vi "pathplan_vertices_send_okkkk.vi"(0 "distance_all":dbl=707.106781186548, 1 "angle_all":cdb[](array[numeric])=[78.5+0.0i, 78.5+0.0i, 78.5+0.0i], 3 "数据发送停止开关":bool, 4 "vertices":dbl[][](array[numeric])=[[0.0, 125.0, 375.0, 500.0], [0.0, 125.0, 375.0, 500.0]], 5 "err":dbl[](array[numeric]), 7 "speed_max":dbl[](array[numeric]), 8 "写入串口":refnum<visa-resource-name>, 9 "distance_send_speed":cdb[](array[numeric])=[0.0+0.0i, 176.776695296637+0.0i, 530.330085889911+0.0i, 707.106781186548+0.0i]) -> (20 "路径规划数据写入缓冲区":string, 21 "stop_all":bool)   [LabVIEW 2016]
uses:
  <vilib>/imath/engines/lvmath2/RunTimeEngine/NodeEndStatement/NIMS_NodeEndStatement_Output.vi
  <instcachedir>/0/NIMS_NodeEndStatement_Output_53EC0D466D134D7ABD903AC30B43404B.lvgen/NIMS_NodeEndStatement_Output_53EC0D466D134D7ABD903AC30B43404B_011.vi
  <vilib>/imath/engines/lvmath2/RunTimeEngine/ErrorHandling/NIMS_Finalize Error.vi
  <vilib>/imath/engines/lvmath2/RunTimeEngine/Managers/WorkSpace/UID Generator.vi
  <vilib>/imath/engines/lvmath2/RunTimeEngine/IndexRead/NIMS M(S).vi
  <instcachedir>/0/NIMS M(S)_B826C018497E4940AE96BD27B540B6FB.lvgen/NIMS M(S)_B826C018497E4940AE96BD27B540B6FB_000.vi
  <vilib>/imath/engines/lvmath2/RunTimeEngine/BuiltInFunctions/abs/NIMS_abs(signed).vi
  <instcachedir>/0/NIMS_abs(signed)_C4FCB8E6058B49B797C7C8D53CA5F6EC.lvgen/NIMS_abs(signed)_C4FCB8E6058B49B797C7C8D53CA5F6EC_000.vi
  <vilib>/imathl/engines/lvmath/Functions/Error Handling/Create Error.vi
  <vilib>/imath/engines/lvmath2/RunTimeEngine/RunTimeType/NIMS_RunTimeType_From StrictType (excl LVString).vi
  <instcachedir>/0/NIMS_RunTimeType_From StrictType (excl LVString)_BBF44FB49F834B71AF7A14CCEDF8BECD.lvgen/NIMS_RunTimeType_From StrictType (excl LVString)_BBF44FB49F834B71AF7A14CCEDF8BECD_000.vi
  <vilib>/imath/engines/lvmath2/RunTimeEngine/LocalVariableDefStatement/MC_LocalVariableDefStatement_Display.vi
  <vilib>/imath/engines/lvmath2/RunTimeEngine/BuiltInFunctions/length/NIMS_length(GM).vi
  <instcachedir>/0/NIMS_length(GM)_47CEC356FCE0482D9BA47DC61C99F2C7.lvgen/NIMS_length(GM)_47CEC356FCE0482D9BA47DC61C99F2C7_000.vi
  <vilib>/imath/engines/lvmath2/RunTimeEngine/RangeToken/NIMS_Range_R2 - Integer.vi
  <instcachedir>/0/NIMS_Range_R2 - Integer_89B873E74E6E489885E44F751DD9C6BF.lvgen/NIMS_Range_R2 - Integer_89B873E74E6E489885E44F751DD9C6BF_000.vi
  <vilib>/imath/engines/lvmath2/RunTimeEngine/CommandStatement/MC_CommandStatement_break.vi
  <vilib>/imath/engines/lvmath2/RunTimeEngine/IndexRead/NIMS M($,S).vi
  <instcachedir>/0/NIMS M($,S)_3E5749BBB62E49528D4765A77F1F6D98.lvgen/NIMS M($,S)_3E5749BBB62E49528D4765A77F1F6D98_000.vi
  <vilib>/imath/engines/lvmath2/RunTimeEngine/ArithmeticOperatorToken/NIMS_ArithmeticOperator_minus.vi
  <instcachedir>/0/NIMS_ArithmeticOperator_minus_E3B65B1D26A44BB184AFDC5B3F458E3D.lvgen/NIMS_ArithmeticOperator_minus_E3B65B1D26A44BB184AFDC5B3F458E3D_002.vi
  <vilib>/imath/engines/lvmath2/RunTimeEngine/ErrorHandling/NIMS_Create Error From Enums.vi
  <vilib>/imath/engines/lvmath2/RunTimeEngine/RowToken/NIMS_RowToken_M_CV.vi
  <instcachedir>/0/NIMS_RowToken_M_CV_FA79F1D1D17D44459F3ED8E09EE8B625.lvgen/NIMS_RowToken_M_CV_FA79F1D1D17D44459F3ED8E09EE8B625_000.vi
  <vilib>/imath/engines/lvmath2/RunTimeEngine/RowToken/NIMS_RowToken_M_M.vi
  <instcachedir>/0/NIMS_RowToken_M_M_968CDE3545E74ACDAEA4B48DE01EEECA.lvgen/NIMS_RowToken_M_M_968CDE3545E74ACDAEA4B48DE01EEECA_004.vi
  <vilib>/imath/engines/lvmath2/RunTimeEngine/RelationalOperatorToken/NIMS_Relational_Operator_Eq.vi
  <instcachedir>/0/NIMS_Relational_Operator_Eq_FD198F059617437A8A02361002FCA645.lvgen/NIMS_Relational_Operator_Eq_FD198F059617437A8A02361002FCA645_006.vi
  <vilib>/imath/engines/lvmath2/RunTimeEngine/BuiltInFunctions/size/NIMS_I32=size(GM,I32).vi
  <instcachedir>/0/NIMS_I32=size(GM,I32)_122058B1B3294FAEA5DC209B92B394E4.lvgen/NIMS_I32=size(GM,I32)_122058B1B3294FAEA5DC209B92B394E4_004.vi
  <instcachedir>/0/NIMS_ArithmeticOperator_minus_E3B65B1D26A44BB184AFDC5B3F458E3D.lvgen/NIMS_ArithmeticOperator_minus_E3B65B1D26A44BB184AFDC5B3F458E3D_003.vi
  <vilib>/imath/engines/lvmath2/RunTimeEngine/BuiltInFunctions/norm/NIMS_norm(GV,DBL).vi
  <instcachedir>/0/NIMS_norm(GV,DBL)_1268AFF3C646412B8C6EA3CE75D09042.lvgen/NIMS_norm(GV,DBL)_1268AFF3C646412B8C6EA3CE75D09042_000.vi
  <vilib>/imath/engines/lvmath2/RunTimeEngine/Managers/SymbolTable/Clear UID.vi
  <instcachedir>/0/NIMS_NodeEndStatement_Output_53EC0D466D134D7ABD903AC30B43404B.lvgen/NIMS_NodeEndStatement_Output_53EC0D466D134D7ABD903AC30B43404B_001.vi
  <instcachedir>/0/NIMS_NodeEndStatement_Output_53EC0D466D134D7ABD903AC30B43404B.lvgen/NIMS_NodeEndStatement_Output_53EC0D466D134D7ABD903AC30B43404B_010.vi
  <instcachedir>/0/NIMS_NodeEndStatement_Output_53EC0D466D134D7ABD903AC30B43404B.lvgen/NIMS_NodeEndStatement_Output_53EC0D466D134D7ABD903AC30B43404B_005.vi
  <vilib>/imath/engines/lvmath2/RunTimeEngine/BuiltInFunctions/length/NIMS_length(GV).vi
  <instcachedir>/0/NIMS_length(GV)_08A3D13377FD4E4B96F5795FBF3698FA.lvgen/NIMS_length(GV)_08A3D13377FD4E4B96F5795FBF3698FA_001.vi
  <vilib>/imath/engines/lvmath2/RunTimeEngine/IndexRead/NIMS V(S).vi
  <instcachedir>/0/NIMS V(S)_0488751826AF41519A22953C041130DC.lvgen/NIMS V(S)_0488751826AF41519A22953C041130DC_003.vi
  <instcachedir>/0/NIMS_abs(signed)_C4FCB8E6058B49B797C7C8D53CA5F6EC.lvgen/NIMS_abs(signed)_C4FCB8E6058B49B797C7C8D53CA5F6EC_002.vi
  <vilib>/imath/engines/lvmath2/RunTimeEngine/VariableToken/NIMS_VariableToken_CondDefined.vi
  <instcachedir>/0/NIMS_VariableToken_CondDefined_06E9DA95BD4D46A6BA55EC651A891960.lvgen/NIMS_VariableToken_CondDefined_06E9DA95BD4D46A6BA55EC651A891960_008.vi
  <vilib>/imath/engines/lvmath/Functions/Error Handling/MergeErrorsWrapper.vi
  <vilib>/imath/engines/lvmath2/RunTimeEngine/Managers/SymbolTable/NIMS_WorkSpace.lvlib
panel:
  in  "distance_now":dbl
  in  "y":dbl[](array[numeric])=[-0.302465]
  in  "x":dbl[](array[numeric])=[0.0274968]
  out "angle_send":dbl[](array[numeric])
  out "vertices_send":dbl[](array[numeric])
  out "speed_send":dbl[](array[numeric])
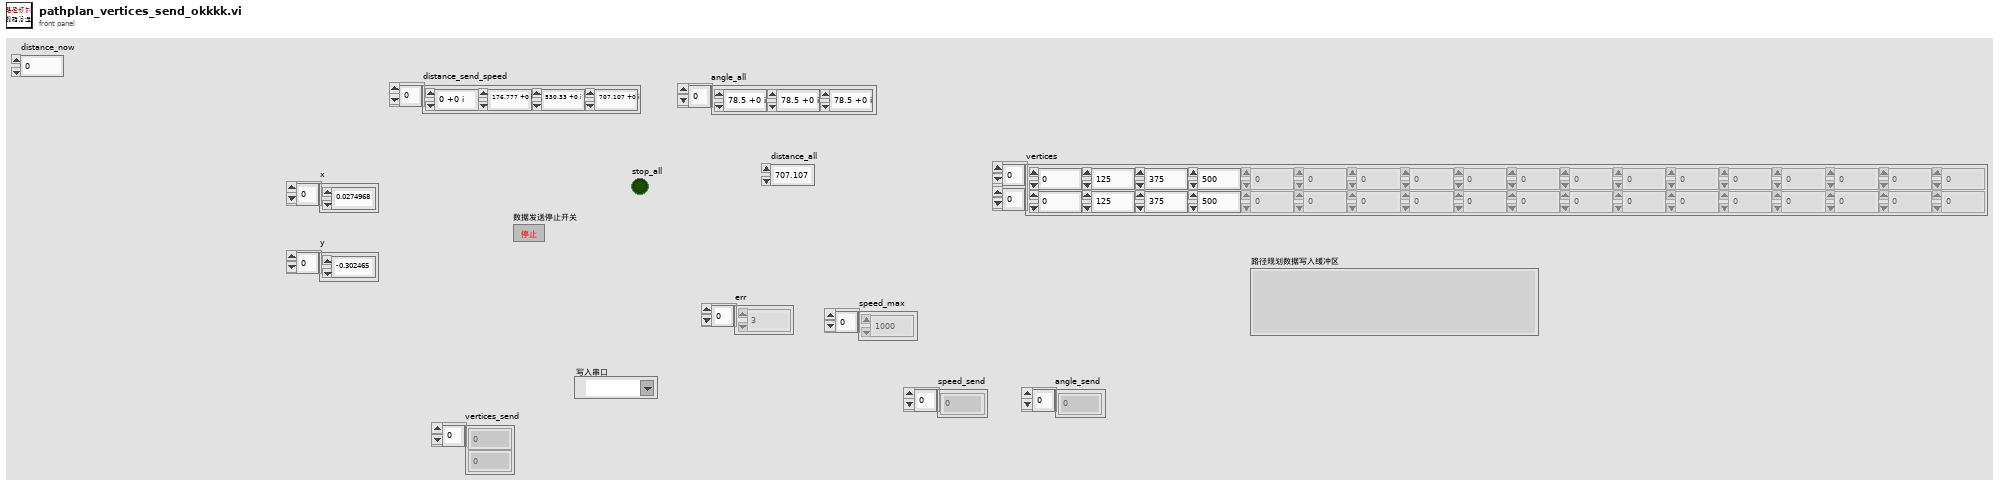
[diagram p1: front panel]
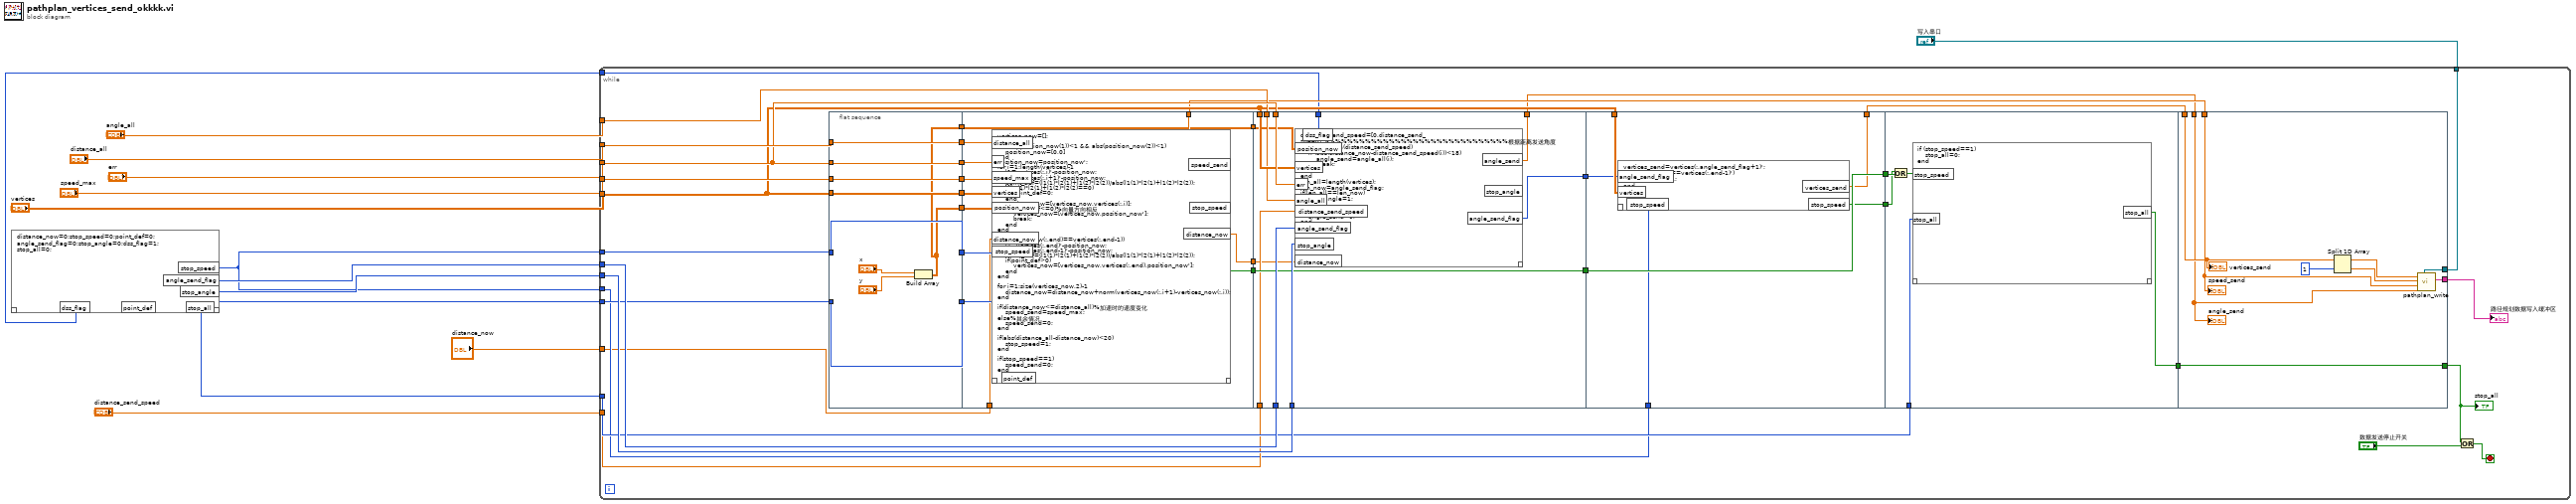
[diagram p0: block diagram]
diagram:
  n1 = mathscript code="distance_now=0;stop_speed=0;point_def=0;\nangle_send_flag=0;stop_angle=0;dss_flag=1;\nstop_all=0;"() -> ("stop_speed"=w2:i32, "angle_send_flag"=w12:i32, "stop_angle"=w13:i32, "stop_all"=w7:i32, "point_def"=w6:i32, "dss_flag"=w5:i32)  [unwired: 1 in, 1 out]
  n2 = while {
    tunnel: "distance_all" -> [w48]
    tunnel: w2 -> [w47]
    tunnel: w13 -> [w46]
    tunnel: w12 -> [w45]
    tunnel: "speed_max" -> [w44]
    tunnel: "err" -> [w43]
    tunnel: "angle_all" -> [w42]
    tunnel: "vertices" -> [w41]
    tunnel: "写入串口" -> [w35]
    tunnel: w7 -> [w40]
    tunnel: w6 -> [w30]
    tunnel: "distance_send_speed" -> [w29]
    tunnel: w5 -> [w27]
    tunnel: w2 -> [w25]
    tunnel: "distance_now" -> [w15]
    stop <- w33 stop-if-true
    n3 = flat-sequence {
      tunnel: w30 -> [w56]
      tunnel: w41 -> [w57]
      tunnel: w44 -> [w58]
      tunnel: w43 -> [w59]
      tunnel: w47 -> [w60]
      tunnel: w48 -> [w61]
      tunnel: [w61] -> w24
      tunnel: [w60] -> w23
      tunnel: [w59] -> w22
      tunnel: [w58] -> w21
      tunnel: [w57] -> w20
      tunnel: [w56] -> w19
      tunnel: [w55] -> w18
      tunnel: [w55] -> w16
      tunnel: [w68] -> w52
      tunnel: [w67] -> w38
      tunnel: [w65] -> w28
      tunnel: w24 -> [w73]
      tunnel: w23 -> [w72]
      tunnel: w22 -> [w71]
      tunnel: w21 -> [w70]
      tunnel: w20 -> [w69]
      tunnel: w19 -> [w66]
      tunnel: w18 -> [w64]
      tunnel: [w63] -> w17
      tunnel: w16 -> [w63]
      tunnel: w15 -> [w62]
      tunnel: w46 -> [w868]
      tunnel: w45 -> [w867]
      tunnel: w43 -> [w866]
      tunnel: w41 -> [w865]
      tunnel: w42 -> [w864]
      tunnel: [w863] -> w51
      tunnel: [w862] -> w50
      tunnel: w52 -> [w862]
      tunnel: [w861] -> w37
      tunnel: w29 -> [w860]
      tunnel: w28 -> [w859]
      tunnel: w27 -> [w858]
      tunnel: w17 -> [w857]
      tunnel: w41 -> [w1090]
      tunnel: w51 -> [w1089]
      tunnel: [w1088] -> w49
      tunnel: w50 -> [w1088]
      tunnel: [w1087] -> w36
      tunnel: [w1086] -> w26
      tunnel: w25 -> [w1085]
      tunnel: w49 -> [w1174]
      tunnel: w40 -> [w1175]
      tunnel: [w1176] -> w39
      tunnel: w26 -> [w1173]
      tunnel: [w1217] -> w34
      tunnel: w39 -> [w1217]
      tunnel: w38 -> [w1213]
      tunnel: w37 -> [w1209]
      tunnel: w36 -> [w1212]
      tunnel: w35 -> [w1211]
      tunnel: [w1210] -> w31
      frame #0 {
        n4 = Build Array("x", "y") -> (w55:dbl[][])
      }
      frame #1 {
        n5 = mathscript code="vertices_now=[];\n\nif (abs(position_now(1))<1 && abs(position_now(2))<1)\n    position_now=[0,0]\nend\nposition_now=position_now';\nfor i=1:length(vertices)-1\n    l1=vertices(:,i)'-position_now;\n    l2=vertices(:,i+1)'-position_now;\n    point_def=(l1(1)*l2(1)+l1(2)*l2(2))/abs(l1(1)*l2(1)+l1(2)*l2(2));\n    if(l1(1)*l2(1)+l1(2)*l2(2)==0)\n        point_def=0;\n    end\n    vertices_now=[vertices_now,vertices(:,i)];\n    if(point_def<=0)%向量方向相反\n        vertices_now=[vertices_now,position_now'];\n        break;\n    end\nend\n\nif(vertices_now(:,end)==vertices(:,end-1))\n    l1=vertices(:,end)'-position_now;\n    l2=vertices(:,end-1)'-position_now;\n    point_def=(l1(1)*l2(1)+l1(2)*l2(2))/abs(l1(1)*l2(1)+l1(2)*l2(2));\n    if(point_def>0)\n        vertices_now=[vertices_now,vertices(:,end),position_now'];\n    end\nend\n\nfor i=1:size(vertices_now,2)-1\n    distance_now=distance_now+norm(vertices_now(:,i+1)-vertices_now(:,i));\nend\n\nif(distance_now<=distance_all)%加速时的速度变化\n    speed_send=speed_max;\nelse%其余情况\n    speed_send=0;\nend\n\nif(abs(distance_all-distance_now)<20)\n    stop_speed=1;\nend\n\nif(stop_speed==1)\n    speed_send=0;\nend"("err"=w71, "speed_max"=w70, "vertices"=w69, "position_now"=w64, "distance_all"=w73, "distance_now"=w62, "stop_speed"=w72, "point_def"=w66) -> ("stop_speed"=w68:bool, "speed_send"=w67:dbl[], "distance_now"=w65:dbl)  [unwired: 1 in, 1 out]
      }
      frame #2 {
        n6 = mathscript code="distance_send_speed=[0,distance_send_speed];%%%%%%%%%%%%%%%%%%%%%%%%%%%%%%%根据距离发送角度\nfor i=1:length(distance_send_speed)\n    if (abs(distance_now-distance_send_speed(i))<18)   \n        angle_send=angle_all(i);\n        break;\n    end\nend\nlen_all=length(vertices);\nlen_now=angle_send_flag;\nif(len_all==len_now)\n    stop_angle=1;\nend\nif (stop_angle==1)\n    angle_send=0;\nend"("err"=w866, "angle_all"=w864, "position_now"=w857, "vertices"=w865, "angle_send_flag"=w867, "stop_angle"=w868, "distance_send_speed"=w860, "distance_now"=w859, "dss_flag"=w858) -> ("angle_send"=w861:dbl[], "angle_send_flag"=w863:i32)  [unwired: 1 in, 2 out]
      }
      frame #3 {
        n7 = mathscript code="vertices_send=vertices(:,angle_send_flag+1)';\nif(vertices_send==vertices(:,end-1)')\n    stop_speed=1;\nend"("angle_send_flag"=w1089, "vertices"=w1090, "stop_speed"=w1085) -> ("vertices_send"=w1087:dbl[], "stop_speed"=w1086:bool)  [unwired: 1 in, 1 out]
      }
      frame #4 {
        n8 = Or(x=w1173, y=w1174) -> (x .or. y?=w1172:bool)
        n9 = mathscript code="if (stop_speed==1)\n    stop_all=0;\nend"("stop_speed"=w1172, "stop_all"=w1175) -> ("stop_all"=w1176:bool)  [unwired: 1 in, 1 out]
      }
      frame #5 {
        n10 = Split 1D Array(array=w1212, index=1 ("索引")) -> (first subarray=w1215:dbl[], second subarray=w1214:dbl[])
        n11 = call "pathplan_write.vi"("VISA资源名称"=w1211, "angle"=w1209, "v"=w1213, "y"=w1214, "x"=w1215) -> ("路径规划数据写入缓冲区"=w1210:string)  [unwired: 6 in]
        "speed_send" <- w1213
        "vertices_send" <- w1212
        "angle_send" <- w1209
      }
    }
    n12 = Or(x=w34, y="数据发送停止开关") -> (x .or. y?=w33:bool)
    "stop_all" <- w34
    "路径规划数据写入缓冲区" <- w31
  }
